vi "F7.vi"(8 "error in":errorcluster, 9 "data":u8[](array[numeric]), 10 "function":u8, 11 "device data model in":refnum<class "Standard Data Model.lvclass">) -> (0 "error out":errorcluster, 1 "data return":u8[](array[numeric]), 2 "function return":u8, 3 "device data model out":refnum<class "Standard Data Model.lvclass">)   [LabVIEW 2013, in "Modbus Library - Advance.lvlib" / "Standard Data Model.lvclass"]
doc: "Executes function code 7"
uses:
  Standard Data Model.lvclass
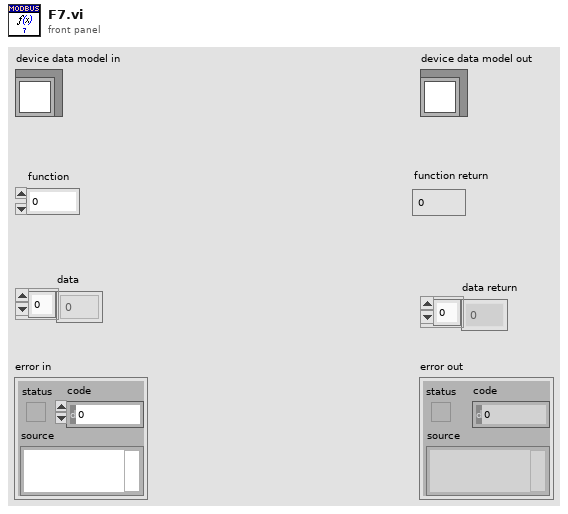
[diagram p1: front panel]
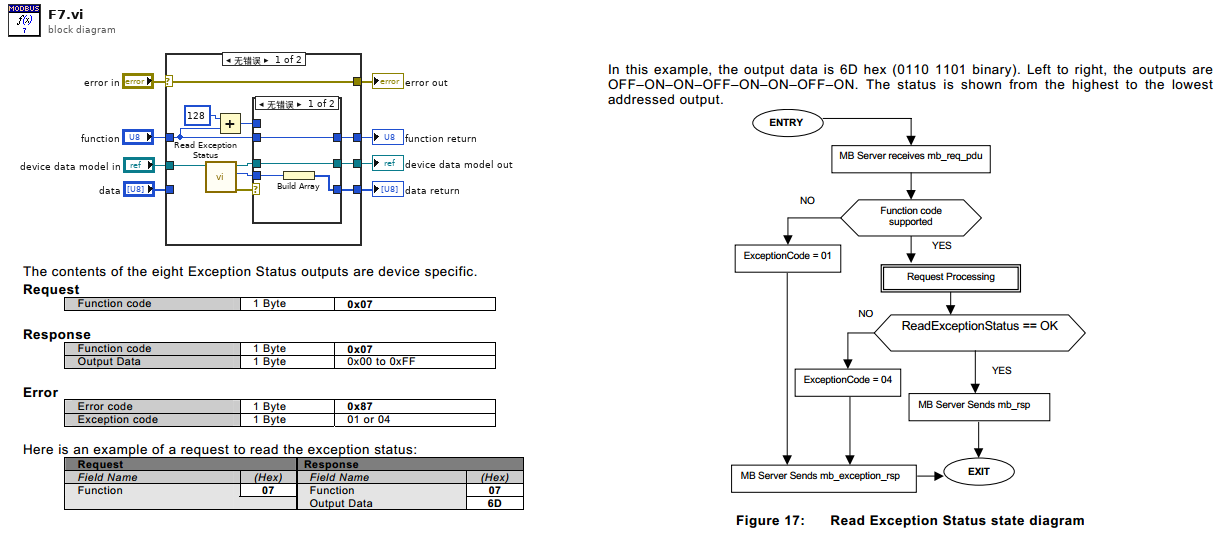
[diagram p0: block diagram]
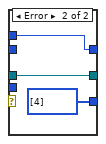
[diagram p2: hidden frame]
diagram:
  n1 = case shown="无错误" "error in" {
    selector: "error in" -> [w19 w30]
    tunnel: [w19 w30] -> w7
    tunnel: [w18 w29] -> w5
    tunnel: "device data model in" -> [w12 w29]
    tunnel: "function" -> [w15 w28]
    tunnel: "data" -> [_ w27]
    tunnel: [w14 w28] -> w2
    tunnel: [w13 w27] -> w1
    frame No Error {
      n2 = call-dynamic "Read Exception Status.vi"("device data model in"=w12) -> ("error out"=w10:errorcluster, "exception status"=w9:u8, "device data model out"=w11:refnum<class "Standard Data Model.lvclass">)  [unwired: 8 in]
      n3 = Add(x=u8 128, y=w15) -> (x+y=w16:u8)
      n4 = case shown="无错误" w10 {
        tunnel: w11 -> [w23 w26]
        tunnel: [w23 w26] -> w18
        tunnel: w16 -> [_ w25]
        tunnel: w15 -> [w22 _]
        tunnel: [w22 w25] -> w14
        tunnel: [w21 u8[] [4]] -> w13
        tunnel: w9 -> [w20 _]
        frame No Error {
          n5 = Build Array(w20) -> (w21:u8[])
        }
        frame Error {
        }
      }
    }
    frame Error {
    }
  }
  "error out" <- w7
  "device data model out" <- w5
  "data return" <- w1
  "function return" <- w2
